vi "VS_OpenWorkspaceMngrRef.vi"(0 "Engine Reference(in)":refnum<k7>, 5 "Sequence File Ref(in)":refnum<k7>, 7 "VeriStand version info":T1={"VeriStand.exe Path"="", "Assembly"="", "Constructor Token"=0, "Module Token"={"GetIWorkspaceToken"=100663761, "GetIStimulusToken"=100663772, "GetIModelManagerToken"=100663768, "GetIProjectToken"=100663780, "RunProjectToken"=100663643, "CloseProjectToken"=100663640, "RunWorkspaceToken"=100663694, "StopWorkspaceToken"=100663695, "SetSingleChannelToken"=100663609, "SetMultipleParametersToken"=100663608, "RunStimulusToken"=100663670, "GetStimulusStateToken"=100663669, "Open WorkspaceToken"=0, "DeployToken"=0, "UndeployToken"=0, "QuitToken"=0}}, 11 "error in":errorcluster, 12 "Step Group":i32(ring) items=["StepGroup_Setup", "StepGroup_Main", "StepGroup_Cleanup"], 13 "Step Index":i32) -> (4 "Engine reference(out)":refnum<k7>, 6 "Sequence File Ref(out)":refnum<k7>, 8 "VeriStand version info (out)":T1={"VeriStand.exe Path"="", "Assembly"="", "Constructor Token"=0, "Module Token"={"GetIWorkspaceToken"=100663761, "GetIStimulusToken"=100663772, "GetIModelManagerToken"=100663768, "GetIProjectToken"=100663780, "RunProjectToken"=100663643, "CloseProjectToken"=100663640, "RunWorkspaceToken"=100663694, "StopWorkspaceToken"=100663695, "SetSingleChannelToken"=100663609, "SetMultipleParametersToken"=100663608, "RunStimulusToken"=100663670, "GetStimulusStateToken"=100663669, "Open WorkspaceToken"=0, "DeployToken"=0, "UndeployToken"=0, "QuitToken"=0}}, 15 "error out":errorcluster)   [LabVIEW 2010]
doc: "This VI creates the VeriStand object reference step in TestStand to access the dotNet API. This VI needs to be called always at the beginning of any VeriStand sequence in TestStand"
uses:
  Ctls/dotNetAssemblyInfo.ctl
  Ctls/VSModuleTokens.ctl
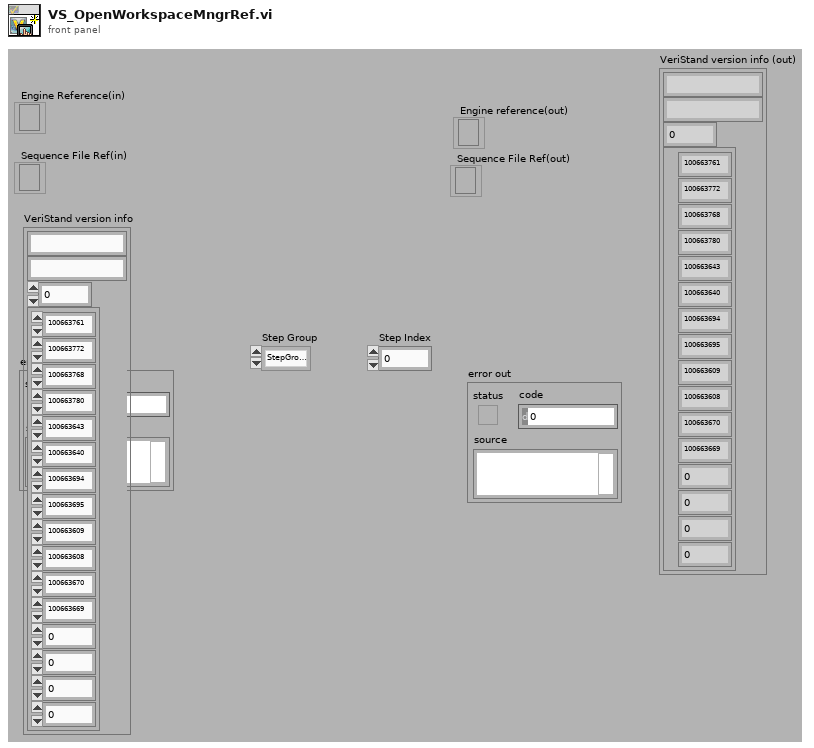
[diagram p1: front panel]
types:
  T1 = typedef "dotNetAssemblyInfo.ctl" = cluster{"VeriStand.exe Path":string, "Assembly":string, "Constructor Token":i32, "Module Token":T2}
  T2 = typedef "VSModuleTokens.ctl" = cluster{"GetIWorkspaceToken":i32, "GetIStimulusToken":i32, "GetIModelManagerToken":i32, "GetIProjectToken":i32, "RunProjectToken":i32, "CloseProjectToken":i32, "RunWorkspaceToken":i32, "StopWorkspaceToken":i32, "SetSingleChannelToken":i32, "SetMultipleParametersToken":i32, "RunStimulusToken":i32, "GetStimulusStateToken":i32, "Open WorkspaceToken":i32, "DeployToken":i32, "UndeployToken":i32, "QuitToken":i32}
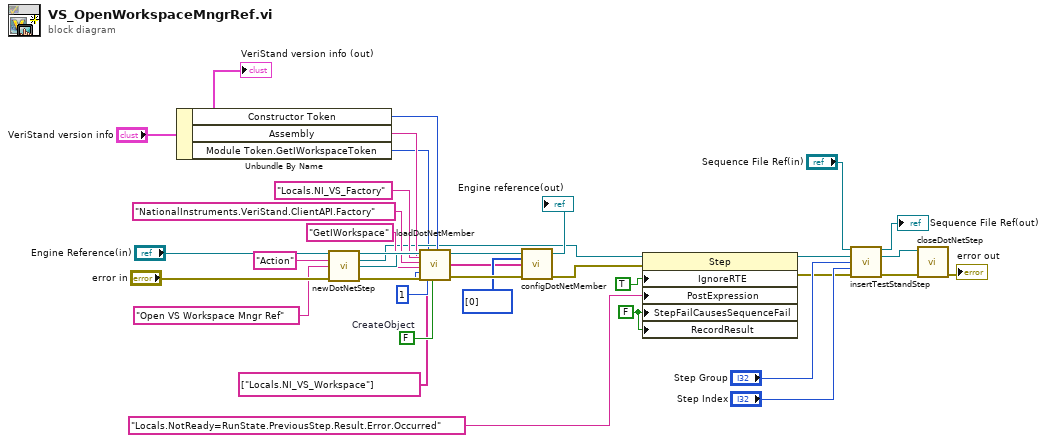
[diagram p0: block diagram]
diagram:
  w2 = FALSE ("StepFailCausesSequenceFail")
  w18 = FALSE  # CreateObject
  n1 = Unbundle By Name("VeriStand version info") -> ("Constructor Token"=w12:i32, "Assembly"=w13:string, "Module Token.GetIWorkspaceToken"=w3:i32)
  n2 = call "newDotNetStep.vi"("Engine reference"="Engine Reference(in)", "stepType"="Action", "Step Name"="Open VS Workspace Mngr Ref", "error in"="error in") -> ("Engine reference(out)"=→"Engine reference(out)":refnum<k7>, "NewStep (out)"=w9:refnum<k7>, "dotNetModule(out)"=w22:refnum<k7>, "error out"=w34:errorcluster)  [unwired: 8 in]
  n3 = call "loadDotNetMember.vi"("dotNetModule"=w22, "Strong Assembly path"=w13, "ClassName"="NationalInstruments.VeriStand.ClientAPI.Factory", "MemberName"="GetIWorkspace", "Member token"=w3, "error in(no error)"=w34, "ClassReference"="Locals.NI_VS_Factory", "Call Member?"=1 ("Call Memeber?"), "CreateObject"=w18, "Constructor Token"=w12) -> ("dotNetModule(out)"=w17:refnum<k7>, "error out"=w16:errorcluster)  [unwired: 8 in]
  n4 = call "configDotNetMember.vi"("dotNetModule"=w17, "Index array"=i32[] [0], "Parameter Value array"=string[] ["Locals.NI_VS_Workspace"], "error in (no error)"=w16) -> ("error out"=w7:errorcluster)  [unwired: 11 in]
  n5 = property class="Step"(reference=w9, error in=w7, "IgnoreRTE"=TRUE, "PostExpression"="Locals.NotReady=RunState.PreviousStep.Result.Error.Occurred" ("ClassReference"), "StepFailCausesSequenceFail"=w2, "RecordResult"=w2) -> (reference out=w5:refnum<k7>, error out=w6:errorcluster)
  n6 = call "insertTestStandStep.vi"("Sequence File Ref"="Sequence File Ref(in)", "Step to insert"=w5, "Step Group"="Step Group", "index"="Step Index", "error out"=w6) -> ("Sequence File Ref(out)"=→"Sequence File Ref(out)":refnum<k7>, "Step to insert (out)"=w33:refnum<k7>, "error out"=w31:errorcluster)  [unwired: 8 in]
  n7 = call "closeDotNetStep.vi"("error in"=w31, "NewStep"=w33) -> ("error out"=→"error out":errorcluster)  [unwired: 9 in]
  "VeriStand version info (out)" <- "VeriStand version info"
